vi "VSI Slave Read Bytes.vi"(9 "WaitTime":i32, 10 "DevIndex":i32, 11 "DevType":i32) -> (1 "function return":i32, 2 "pBytesNum":i32, 3 "pReadData":u8[](array[numeric]))   [LabVIEW 2010, in "ControlSPI.lvlib"]
doc: "int WINAPI VSI_SlaveReadBytes(int DevType,int DevIndex,unsigned char *pReadData,int *pBytesNum,int WaitTime);"
uses:
  ControlSPI.lvlib
  ControlSPI/Ginkgo_Driver.dll
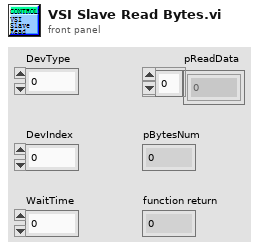
[diagram p1: front panel]
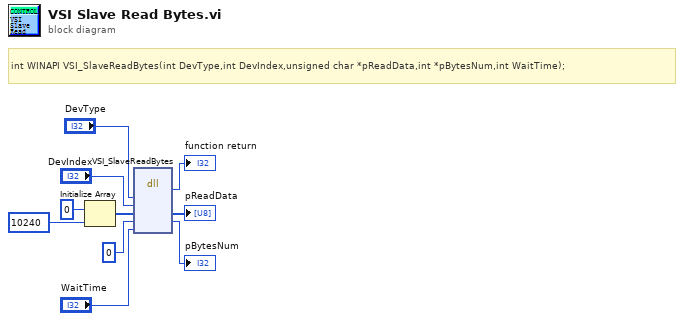
[diagram p0: block diagram]
diagram:
  # "int WINAPI VSI_SlaveReadBytes(int DevType,int DevIndex,unsigned char *pReadData,int *pBytesNum,int WaitTime);"
  n1 = Initialize Array(u8 0 ("element"), 10240 ("dimension size")) -> (w7:u8[])
  n2 = dll-call lib="E:/Project/vt_ginkgo/truck/Ginkgo Driver/vs2010/Ginkgo_USB-I2C&SPI&CAN_API_v2.0.3.3/lib/labview_32bit/ControlSPI/Ginkgo_Driver.*" fn="VSI_SlaveReadBytes"("DevType"="DevType", "DevIndex"="DevIndex", "pReadData"=w7, "pBytesNum"=0, "WaitTime"="WaitTime") -> (→"function return":i32, "pReadData"=→"pReadData":u8[], "pBytesNum"=→"pBytesNum":i32)  [unwired: 6 in, 2 out]
